vi "SetDefaults.vi"(8 "error in (no error)":errorcluster, 11 "ExampleParser in":refnum<class "ExampleParser.lvclass">) -> (0 "error out":errorcluster, 3 "ExampleParser out":refnum<class "ExampleParser.lvclass">)   [LabVIEW 2022 SP3, in "ArgumentParser.lvlib" / "ExampleParser.lvclass"]
uses:
  ExampleParser.lvclass
  C:/Users/jakub/repos/gh/sw4sys/lv-argument-parser/ArgumentParser/Source/ArgumentParser/ArgumentParser.lvclass
  ArgumentParser/ArgumentParser.lvclass/ArgumentParser.ctl
  ArgumentParser/Write ParserPath.vi
  ArgumentParser/ArgumentParser.lvclass
  ExampleParser.lvclass/ExampleParser.ctl
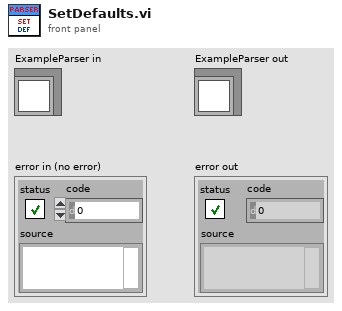
[diagram p1: front panel]
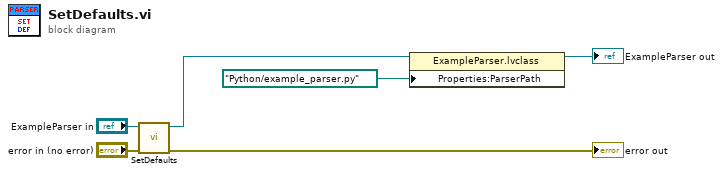
[diagram p0: block diagram]
diagram:
  n1 = call-parent "SetDefaults.vi"("error in (no error)"="error in (no error)", "ArgparseWrapper in"="ExampleParser in") -> ("error out"=→"error out":errorcluster, "ArgparseWrapper out"=w3:refnum<class "ExampleParser.lvclass">)  [unwired: 8 in]
  n2 = property class="ExampleParser.lvclass"(reference=w3, "Properties:ParserPath"=path "Python/example_parser.py" ("ParserPath")) -> (reference out=→"ExampleParser out":refnum<class "ExampleParser.lvclass">)  [unwired: 1 in, 1 out]
